vi "Add Palette Item.vi"(8 "error in (no error)":errorcluster, 9 "Group (From Step Type)":string, 10 "Step Type Name":string, 11 "InsertionPalettePanel in":refnum<class "InsertionPalettePanel.lvclass">) -> (0 "error out":errorcluster, 3 "InsertionPalettePanel out":refnum<class "InsertionPalettePanel.lvclass">)   [LabVIEW 2020, in "TSnax UI.lvlib" / "InsertionPalettePanel.lvclass"]
uses:
  InsertionPalettePanel.lvclass
  InsertionPalettePanel.lvclass/InsertionPalettePanel.ctl
  StepTypeMenuItem/StepTypeMenuItem.lvclass
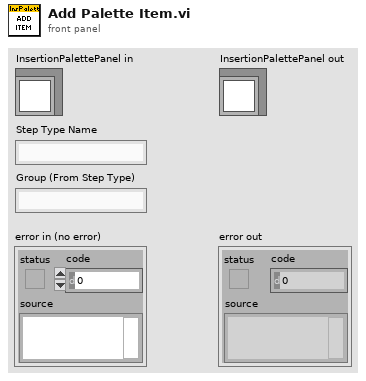
[diagram p1: front panel]
types:
  T1 = typedef "TSnax UI.lvlib/InsertionPalettePanel.lvclass/Ref Data.ctl" = cluster{"Menu Items":map{string, refnum<class "StepTypeMenuItem.lvclass">}}
  T2 = map{string, refnum<class "StepTypeMenuItem.lvclass">}
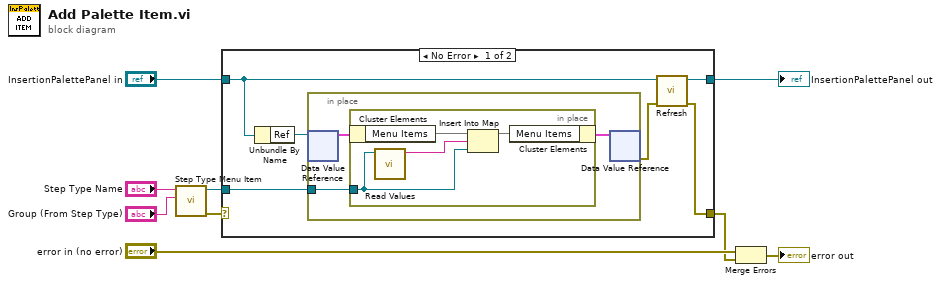
[diagram p0: block diagram]
diagram:
  n1 = call "Step Type Menu Item.vi"("Group (From Step)"="Group (From Step Type)", "Step Type Name"="Step Type Name") -> ("error out"=w2:errorcluster, "StepTypeMenuItem"=w1:refnum<class "StepTypeMenuItem.lvclass">)  [unwired: 8 in]
  n2 = case shown="No Error" w2 {
    selector: w2 -> [_ w24]
    tunnel: "InsertionPalettePanel in" -> [w14 w23]
    tunnel: [w12 w23] -> w7
    tunnel: [w11 w24] -> w5
    tunnel: w1 -> [w10 _]
    frame No Error {
      n3 = Unbundle By Name(w14) -> ("Ref"=w15:refnum<data-value>)
      n4 = in-place {
        in-place-border: w10 -> [w16]
        n5 = in-place-dvr #1(w15) -> (w18:T1)  [unwired: 1 out]
        n6 = in-place {
          in-place-border: w16 -> [w19]
          n7 = in-place-cluster #2(w18) -> ("Menu Items"=w22:T2)
          n8 = call "Read Values.vi"("StepTypeMenuItem in"=w19) -> ("Step Type"=w20:string)  [unwired: 8 in, 2 out]
          n9 = Insert Into Map(map in=w22, key=w20, value=w19) -> (map out=w21:T2)  [unwired: 2 out]
          n10 = in-place-cluster #2("Menu Items"=w21) -> (w17:T1)
        }
        n11 = in-place-dvr #1(w17) -> (w13:errorcluster)  [unwired: 1 out]
      }
      n12 = call "Refresh.vi"("error in (no error)"=w13, "InsertionPalettePanel in"=w14) -> ("error out"=w11:errorcluster, "InsertionPalettePanel out"=w12:refnum<class "InsertionPalettePanel.lvclass">)  [unwired: 8 in]
    }
    frame Error {
    }
  }
  "InsertionPalettePanel out" <- w7
  n13 = Merge Errors("error in (no error)", w5) -> (→"error out":errorcluster)
